vi "Set Instrument Addon Name_ex.vi"() -> ()   [LabVIEW 2019]
uses:
  <vilib>/NI VeriStand/Custom Device API/Custom Device Item Ref.ctl
  Scripting API/Scripting API.lvlib
  <vilib>/NI VeriStand/Custom Device API/Custom Device API.lvlib
panel:
  out "instrument addon refnum out":T1=18446744073709551615 format="%.0x"
  out "error out":errorcluster
  in  "instrument addon refnum in":T1=18446744073709551615 format="%.0x"
  in  "name":string
  in  "error in (no error)":errorcluster
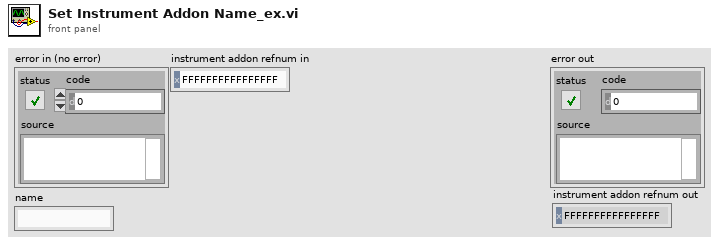
[diagram p1: front panel]
types:
  T1 = typedef "Custom Device API.lvlib/Custom Device Item Ref.ctl" = u64
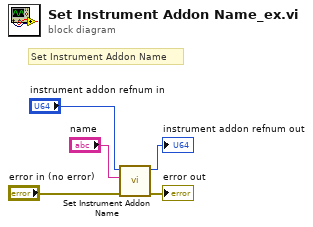
[diagram p0: block diagram]
diagram:
  # "Set Instrument Addon Name"
  n1 = call "Set Instrument Addon Name.vi"("error in (no error)"="error in (no error)", "name"="name", "instrument addon refnum in"="instrument addon refnum in") -> ("error out"=→"error out":errorcluster, "instrument addon refnum out"=→"instrument addon refnum out":T1)  [unwired: 7 in]
